vi "status message.vi"(0 "state":string, 1 "message":string, 3 "error in (no error)":errorcluster, 4 "name (unnamed)":string) -> (10 "error out":errorcluster)   [LabVIEW 2019]
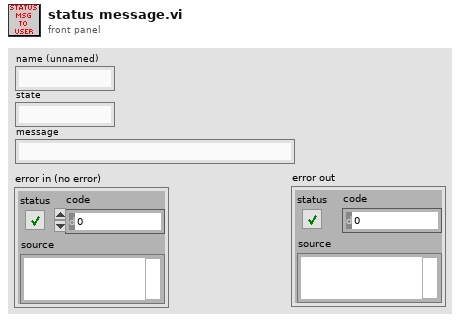
[diagram p1: front panel]
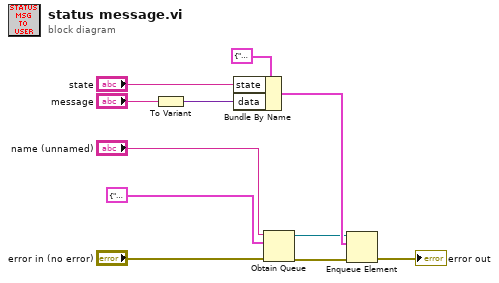
[diagram p0: block diagram]
diagram:
  n1 = To Variant(anything="message") -> (Variant=w4:variant)
  n2 = Bundle By Name(cluster=cluster{"state":string, "data":variant} {"state"="", "data"=variant} ("element"), "state"="state", "data"=w4) -> (w10:cluster{"state":string, "data":variant})
  n3 = Obtain Queue(name (unnamed)="name (unnamed)", element data type=cluster{"state":string, "data":variant} {"state"="", "data"=variant} ("element"), error in (no error)="error in (no error)") -> (queue out=w8:refnum<queue>, error out=w9:errorcluster)  [unwired: 2 in, 1 out]
  n4 = Enqueue Element(queue=w8, element=w10, error in (no error)=w9) -> (error out=→"error out":errorcluster)  [unwired: 1 in, 2 out]
